vi "mymodule.vi"() -> ()   [LabVIEW 2018]
uses:
  <vilib>/Enthought/Python Integration Toolkit/api/Unpack Double.vi
  <vilib>/Enthought/Python Integration Toolkit/api/Unpack Int.vi
  <vilib>/Enthought/Python Integration Toolkit/Python Integration Toolkit.lvlib
panel:
  out "数组":i32[](array[numeric])
  out "数值 2":dbl
  in  "数值":dbl
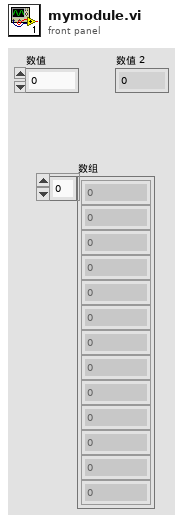
[diagram p1: front panel]
types:
  T1 = typedef "Python Integration Toolkit.lvlib/Session ID.ctl" = u64
  T2 = typedef "Python Integration Toolkit.lvlib/Python Objects.ctl" = variant
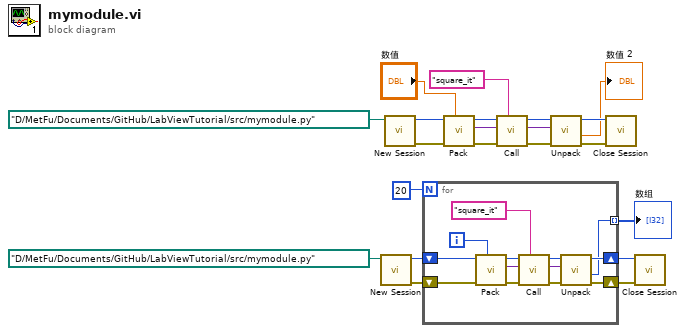
[diagram p0: block diagram]
diagram:
  n1 = call <vilib>:"New Session.vi"("Path to Python Module (.py File)"=path "D:/MetFu/Documents/GitHub/LabViewTutorial/src/mymodule.py") -> ("error out"=w4:errorcluster, "Session ID out"=w5:T1)  [unwired: 9 in]
  n2 = call <vilib>:"New Session.vi"("Path to Python Module (.py File)"=path "D:/MetFu/Documents/GitHub/LabViewTutorial/src/mymodule.py") -> ("error out"=w18:errorcluster, "Session ID out"=w21:T1)  [unwired: 9 in]
  n3 = for {
    N: 20 -> [_]
    shift-right: [w26] -> w2
    shift-left: w5 -> [w25]
    shift-right: [w23] -> w3
    shift-left: w4 -> [w24]
    tunnel: [w22] -> w1 mode=indexing
    i -> [w27]
    n4 = call <vilib>:"Pack.vi"("Argument"=w27, "error in (no error)"=w24, "Session ID"=w25) -> ("error out"=w33:errorcluster, "Python Object References Out"=w29:T2, "Session ID out"=w30:T1)  [unwired: 6 in]
    n5 = call <vilib>:"Call.vi"("Function or Method Name"="square_it", "error in (no error)"=w33, "Python Object References In"=w29, "Session ID"=w30) -> ("error out"=w32:errorcluster, "Python Object References Out"=w31:T2, "Session ID out"=w34:T1)  [unwired: 5 in]
    n6 = call-poly <vilib>:"Unpack.vi"("error in (no error)"=w32, "Python Object References In"=w31, "Session ID"=w34) -> ("error out"=w23:errorcluster, "Value"=w22:i32, "Session ID out"=w26:T1)  [unwired: 5 in, 1 out]
  }
  "数组" <- w1
  n7 = call <vilib>:"Pack.vi"("Argument"="数值", "error in (no error)"=w18, "Session ID"=w21) -> ("error out"=w17:errorcluster, "Python Object References Out"=w8:T2, "Session ID out"=w9:T1)  [unwired: 6 in]
  n8 = call <vilib>:"Call.vi"("Function or Method Name"="square_it", "error in (no error)"=w17, "Python Object References In"=w8, "Session ID"=w9) -> ("error out"=w16:errorcluster, "Python Object References Out"=w10:T2, "Session ID out"=w20:T1)  [unwired: 5 in]
  n9 = call-poly <vilib>:"Unpack.vi"("error in (no error)"=w16, "Python Object References In"=w10, "Session ID"=w20) -> ("error out"=w15:errorcluster, "Value"=→"数值 2":dbl, "Session ID out"=w19:T1)  [unwired: 5 in, 1 out]
  n10 = call <vilib>:"Close Session.vi"("error in (no error)"=w15, "Session ID"=w19) -> ()  [unwired: 9 in, 1 out]
  n11 = call <vilib>:"Close Session.vi"("error in (no error)"=w3, "Session ID"=w2) -> ()  [unwired: 9 in, 1 out]
